vi "Channel3Conv.vi"(8 "error in (no error)":errorcluster, 11 "Multi Channel ADC in":refnum<class "Multi Channel ADC.lvclass">) -> (0 "error out":errorcluster, 2 "Channel 3 U8 Array":u8[](array[numeric]), 3 "Multi Channel ADC out":refnum<class "Multi Channel ADC.lvclass">)   [LabVIEW 2023, in "Multi Channel ADC.lvclass"]
uses:
  Multi Channel ADC.lvclass
  C:/Users/santharu.subramanian/Documents/ADC_SDLC/ADC_SDLC/Adc/Classes/Conversion/Conversion.lvclass
  <vilib>/numeric/Random Number (Range) U64.vi
  <vilib>/numeric/sub_Random U32.vi
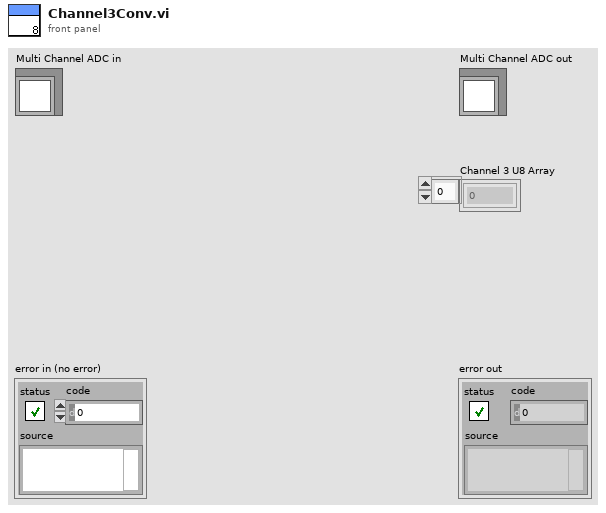
[diagram p1: front panel]
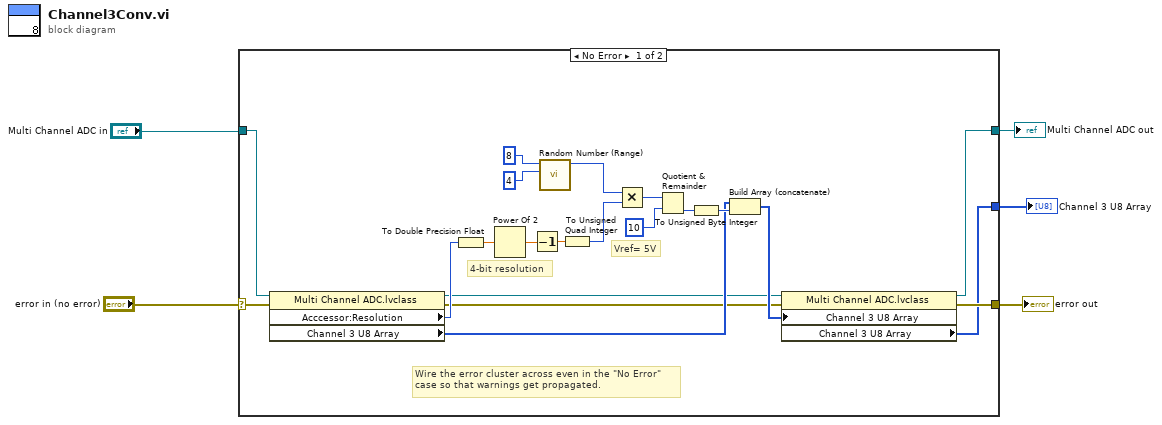
[diagram p0: block diagram]
diagram:
  n1 = case shown="No Error" "error in (no error)" {
    selector: "error in (no error)" -> [w12 w28]
    tunnel: [w8 w28] -> w3
    tunnel: [w7 w27] -> w2
    tunnel: "Multi Channel ADC in" -> [w13 w27]
    tunnel: [w6 _] -> w1
    frame No Error {
      # "Vref= 5V"
      # "4-bit resolution"
      # "Wire the error cluster across even in the \"No Error\"\ncase so that warnings get propagated."
      n2 = property class="Multi Channel ADC.lvclass"(reference=w13, error in=w12) -> (reference out=w9:refnum<class "Multi Channel ADC.lvclass">, error out=w10:errorcluster, "Acccessor:Resolution"=w15:i32, "Channel 3 U8 Array"=w14:u8[])
      n3 = To Double Precision Float(number=w15) -> (double precision float=w19:dbl)
      n4 = Power Of 2(x=w19) -> (2^x=w21:dbl)
      n5 = Decrement(x=w21) -> (x-1=w26:dbl)
      n6 = call-poly <vilib>:"Random Number (Range).vi"("lower bound (0)"=u64 4, "upper bound (100)"=u64 8) -> ("number"=w16:u64)  [unwired: 9 in]
      n7 = To Unsigned Quad Integer(1:w26) -> (0:w20:u64)
      n8 = Multiply(x=w16, y=w20) -> (x*y=w24:u64)
      n9 = Quotient & Remainder(x=w24, y=u64 10 ("upper bound (100)")) -> (floor(x/y)=w23:u64)  [unwired: 1 out]
      n10 = To Unsigned Byte Integer(number=w23) -> (unsigned 8bit integer=w22:u8)
      n11 = Build Array (concatenate)(w14, w22) -> (w11:u8[])
      n12 = property class="Multi Channel ADC.lvclass"(reference=w9, error in=w10, "Channel 3 U8 Array"=w11) -> (reference out=w7:refnum<class "Multi Channel ADC.lvclass">, error out=w8:errorcluster, "Channel 3 U8 Array"=w6:u8[])
    }
    frame Error {
    }
  }
  "error out" <- w3
  "Multi Channel ADC out" <- w2
  "Channel 3 U8 Array" <- w1
